vi "Write VISA resource name.vi"(8 "error in (no error)":errorcluster, 10 "VISA resource name":refnum<visa-resource-name>, 11 "ArduinoControl in":refnum<class "ArduinoControl.lvclass">) -> (0 "error out":errorcluster, 3 "ArduinoControl out":refnum<class "ArduinoControl.lvclass">)   [LabVIEW 2019, in "ArduinoControl.lvclass"]
uses:
  ArduinoControl.lvclass
  ArduinoControl.lvclass/ArduinoControl.ctl
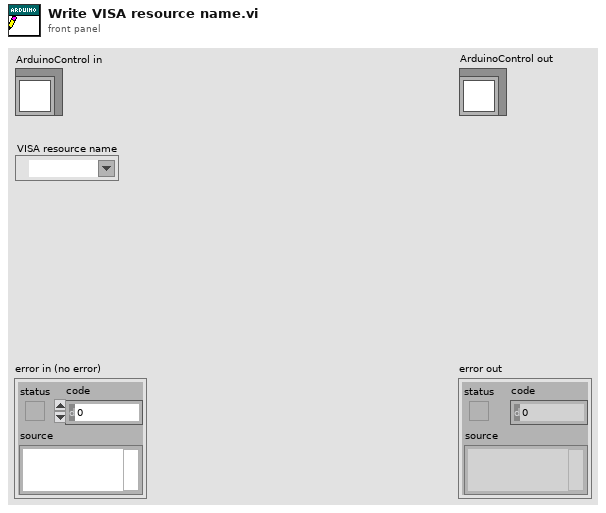
[diagram p1: front panel]
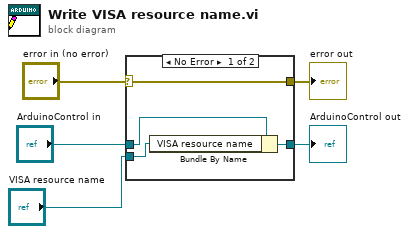
[diagram p0: block diagram]
diagram:
  n1 = case shown="No Error" "error in (no error)" {
    selector: "error in (no error)" -> [w9 w10]
    tunnel: [w9 w10] -> w4
    tunnel: [w7 w11] -> w2
    tunnel: "ArduinoControl in" -> [w6 w11]
    tunnel: "VISA resource name" -> [w8 _]
    frame No Error {
      n2 = Bundle By Name(cluster=w6, "VISA resource name"=w8) -> (w7:refnum<class "ArduinoControl.lvclass">)
    }
    frame Error {
    }
  }
  "error out" <- w4
  "ArduinoControl out" <- w2
